vi "ExTestCustomChip.vi"() -> ()   [LabVIEW 2010]
panel:
  out "Boolean":bool
  out "x Size":u32
  out "x post":u32
  out "x pre":u32
  out "y Size":u32
  out "y post":u32
  out "y pre":u32
  in  "Software Accumulation":u32=1 min=1 step=1
  in  "Intensifier":bool
  in  "Temperature":dbl=-10.0 format="%.2f"
  in  "Exposure":dbl min=0.0 step=1e-06 format="%.5f"
  in  "stop":bool
  in  "Store":bool
  out "error out":errorcluster
  in  "error in (no error)":errorcluster
  # "ExTestCustomChip:\nThis example only works with cameras with circualar\n buffer capability. Get current pre-post strip and setup\n to do complete scan of whole CCD including dummies.\nThis example well only work with Princeton Instruments\nCamreas, not Photometrics"
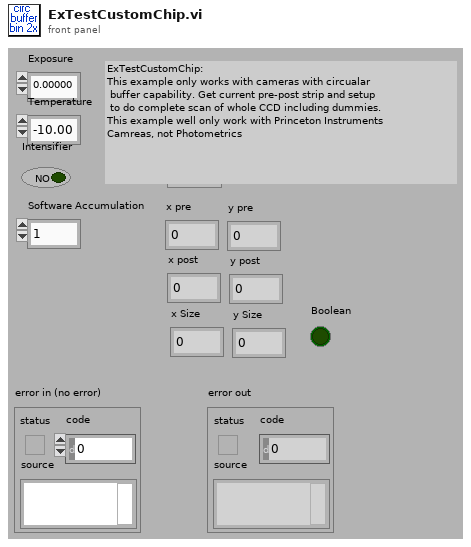
[diagram p1: front panel]
types:
  T1 = cluster{"Pre Y":u32, "Post Y":u32, "Parallel (Y) Size":u32, "Pre X":u32, "Post X":u32, "Serial (X) Size":u32}
  T2 = cluster{"acquire focus mode":u32, "Exposure":dbl, "Number of Images":u32, "Software Accumulation":u32}
  T3 = cluster{"Camera Handle":u32, "Pulser Handle":u32, "File Handle":u32, "Display Handle":u32, "Image Handle":u32}
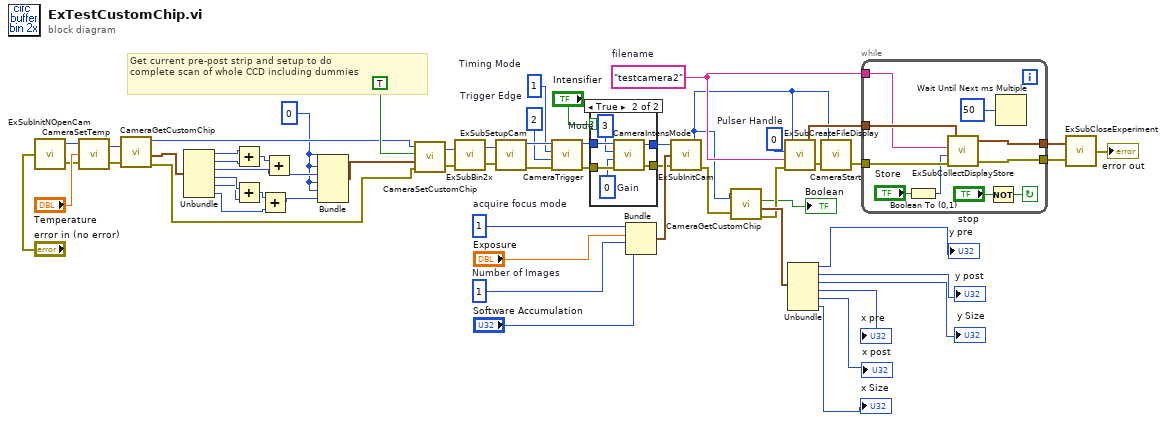
[diagram p0: block diagram]
diagram:
  w3 = 0
  w42 = u32 0  # Pulser Handle
  w43 = u32 1  # Timing Mode
  w44 = u32 2  # Trigger Edge
  w46 = u32 1  # acquire focus mode
  w45 = u32 1  # Number of Images
  w59 = "testcamera2"  # filename
  # "Get current pre-post strip and setup to do \ncomplete scan of whole CCD including dummies"
  n1 = call "ExSubInitNOpenCam.vi"("error in (no error)"="error in (no error)") -> ("Camera Handle"=w35:u32, "error out"=w33:errorcluster)
  n2 = call <userlib>:"CameraSetTemp.vi"("error in (no error)"=w33, "Temperature"="Temperature", "Camera Handle"=w35) -> ("error out"=w17:errorcluster, "Camera Handle"=w16:u32)
  n3 = call <userlib>:"CameraGetCustomChip.vi"("Camera Handle"=w16, "error in (no error)"=w17) -> ("Camera Handle"=w14:u32, "CameraGetCustomChip"=w1:T1, "error out"=w15:errorcluster)  [unwired: 1 out]
  n4 = Unbundle(w1) -> ("Pre Y"=w13:u32, "Post Y"=w12:u32, "Parallel (Y) Size"=w10:u32, "Pre X"=w9:u32, "Post X"=w8:u32, "Serial (X) Size"=w6:u32)
  n5 = Add(x=w13, y=w12) -> (x+y=w11:u32)
  n6 = Add(x=w9, y=w8) -> (x+y=w7:u32)
  n7 = Add(x=w7, y=w6) -> (x+y=w4:u32)
  n8 = Add(x=w11, y=w10) -> (x+y=w5:u32)
  n9 = Bundle(w3, w3, w5, w3, w3, w4) -> (w2:cluster{i32, i32, u32, i32, i32, u32})  [unwired: 1 in]
  n10 = call <userlib>:"CameraSetCustomChip.vi"("error in (no error)"=w15, "Custom Chip Settings"=w2, "Enable/Disable Custom Chip"=TRUE, "Camera Handle"=w14) -> ("error out"=w20:errorcluster, "Camera Handle"=w19:u32)
  n11 = call "ExSubBin2x.vi"("error in (no error)"=w20, "Camera Handle"=w19) -> ("error out"=w32:errorcluster, "Camera Handle"=w47:u32)
  n12 = call "ExSubSetupCam.vi"("error in (no error)"=w32, "Camera Handle"=w47) -> ("error out"=w50:errorcluster, "Camera Handle"=w51:u32)
  n13 = call <userlib>:"CameraTrigger.vi"("error in"=w50, "Trigger Edge"=w44, "Timing Mode"=w43, "Camera Handle"=w51) -> ("error out"=w39:errorcluster, "Camera Handle"=w41:u32)
  n14 = case shown="True" "Intensifier" {
    tunnel: w41 -> [w61 w67]
    tunnel: [w61 w66] -> w40
    tunnel: w39 -> [w60 w65]
    tunnel: [w60 w64] -> w38
    frame False {
    }
    frame True {
      w62 = u32 0  # Gain
      w63 = u32 3  # Mode
      n15 = call <userlib>:"CameraIntensMode.vi"("error in"=w65, "Intensifier Gain"=w62, "Mode"=w63, "Camera Handle"=w67) -> ("error out"=w64:errorcluster, "Camera Handle"=w66:u32)
    }
  }
  n16 = Bundle("acquire focus mode"=w46, "Exposure"="Exposure", "Number of Images"=w45, "Software Accumulation"="Software Accumulation") -> (w56:T2)  [unwired: 1 in]
  n17 = call "ExSubInitCam.vi"("error in (no error)"=w38, "Camera Information"=w56, "Camera Handle"=w40) -> ("error out"=w23:errorcluster, "Camera Handle"=w31:u32)
  n18 = call <userlib>:"CameraGetCustomChip.vi"("Camera Handle"=w31, "error in (no error)"=w23) -> ("Custum chip Enable/Disable status"=→"Boolean":bool, "CameraGetCustomChip"=w30:T1, "error out"=w22:errorcluster)  [unwired: 1 out]
  n19 = call "ExSubCreateFileDisplay.vi"("error in (no error)"=w22, "File and Display Name"=w59, "Pulser Handle"=w42, "Camera Handle"=w31) -> ("error out"=w48:errorcluster, "Handles Out"=w55:T3)
  n20 = Unbundle(w30) -> ("Pre Y"=→"y pre":u32, "Post Y"=→"y post":u32, "Parallel (Y) Size"=→"y Size":u32, "Pre X"=→"x pre":u32, "Post X"=→"x post":u32, "Serial (X) Size"=→"x Size":u32)
  n21 = call <userlib>:"CameraStart.vi"("error in"=w48, "Camera Handle"=w31) -> ("error out"=w49:errorcluster)  [unwired: 1 out]
  n22 = while {
    tunnel: w55 -> [w76]
    tunnel: w49 -> [w75]
    tunnel: w59 -> [w68]
    tunnel: [w73] -> w53
    tunnel: [w74] -> w54
    stop <- w71 continue-if-true
    n23 = Boolean To (0,1)(Boolean="Store") -> (0, 1=w69:i16)
    n24 = call "ExSubCollectDisplayStore.vi"("error in (no error)"=w75, "Store flag"=w69, "Display Title"=w68, "Handle Cluster"=w76) -> ("error out"=w73:errorcluster, "Handle Cluster Out"=w74:T3)  [unwired: 1 out]
    n25 = Not(x="stop") -> (.not. x?=w71:bool)
    n26 = Wait Until Next ms Multiple(millisecond multiple=u32 50) -> ()  [unwired: 1 out]
  }
  n27 = call "ExSubCloseExperiment.vi"("error in (no error)"=w53, "Handles In"=w54) -> ("error out"=→"error out":errorcluster)
